vi "Real Matrix Rank.vi"(2 "tolerance":dbl=-1.0 format="%.2f", 3 "Input Matrix":T1) -> (0 "error":i32, 1 "rank":i32)   [LabVIEW 2018, in "NI_AALPro.lvlib"]
doc: "Computes the rank of <B>Input Matrix</B>. Wire data to the <B>Input Matrix</B> input to determine the polymorphic instance to use or manually select the instance."
uses:
  <vilib>/Analysis/NI_AALPro.lvlib
  RealMatrix.ctl
  <resource>/lvanlys.dll
  NI_Matrix.lvlib
panel:
  # "Matrix Rank"
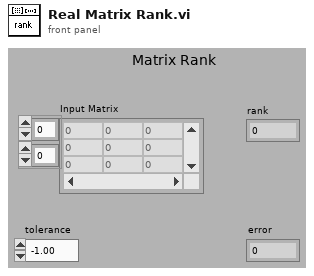
[diagram p1: front panel]
types:
  T1 = typedef "NI_Matrix.lvlib/RealMatrix.ctl" = dbl[][]
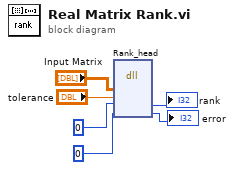
[diagram p0: block diagram]
diagram:
  n1 = dll-call lib="C:/Program Files (x86)/National Instruments/LabVIEW 2018/resource/lvanlys.*" fn="Rank_head"("Input Matrix"="Input Matrix", "tolerance"="tolerance", 0, 0) -> (→"rank":i32, →"error":i32)  [unwired: 6 in, 2 out]
